vi "ClientGlobalCY.vi"() -> ()   [LabVIEW 2014]
panel:
  in  "connection ID":refnum<k5>
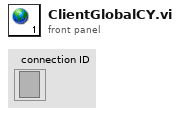
[diagram p1: front panel]
diagram:
